vi "Get Provided Interface and Service Class.vi"(8 "error in":errorcluster, 11 "instrument in":refnum<class "Instrument.lvclass">) -> (0 "error out":errorcluster, 1 "service class":string, 2 "provided interface":string, 3 "instrument out":refnum<class "Instrument.lvclass">)   [LabVIEW 2020, in "MeasurementLink 34401.lvlib" / "Instrument.lvclass"]
uses:
  Instrument.lvclass
  Instrument.lvclass/Instrument.ctl
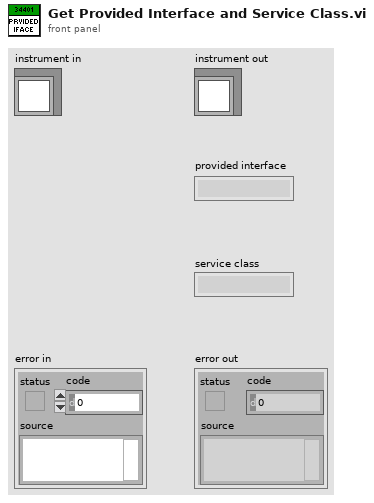
[diagram p1: front panel]
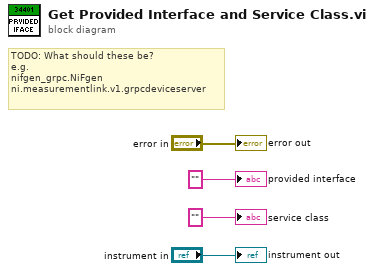
[diagram p0: block diagram]
diagram:
  # "TODO: What should these be?\ne.g.\nnifgen_grpc.NiFgen\nni.measurementlink.v1.grpcdeviceserver"
  "error out" <- "error in"
  "instrument out" <- "instrument in"
  "provided interface" <- "" ("provided interface")
  "service class" <- "" ("service_class")
